vi "euclidean_distance_double.vi"(8 "Point 2 Y":dbl, 9 "Point 2 X":dbl, 10 "Point 1 Y":dbl, 11 "Point 1 X":dbl) -> (3 "Distance":dbl)   [LabVIEW 2019]
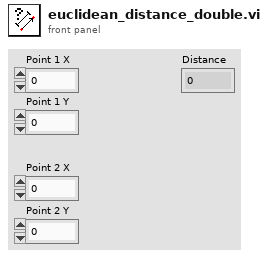
[diagram p1: front panel]
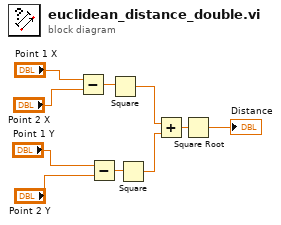
[diagram p0: block diagram]
diagram:
  n1 = Subtract(x="Point 1 X", y="Point 2 X") -> (x-y=w10:dbl)
  n2 = Subtract(x="Point 1 Y", y="Point 2 Y") -> (x-y=w9:dbl)
  n3 = Square(x=w10) -> (x^2=w8:dbl)
  n4 = Square(x=w9) -> (x^2=w7:dbl)
  n5 = Add(x=w8, y=w7) -> (x+y=w6:dbl)
  n6 = Square Root(x=w6) -> (sqrt(x)=→"Distance":dbl)
